vi "Paths to String with Commas.vi"(10 "Paths":string[](array[string])) -> (1 "Columns":string, 2 "Table":string)   [LabVIEW 2019, in "LV-Data.PGSQL.lvclass"]
uses:
  LV-Data.PGSQL.lvclass
  babc5d78-c446-43dc-b590-f0a1f3a79644.vi
panel:
  out "error out":errorcluster
  in  "error in":errorcluster
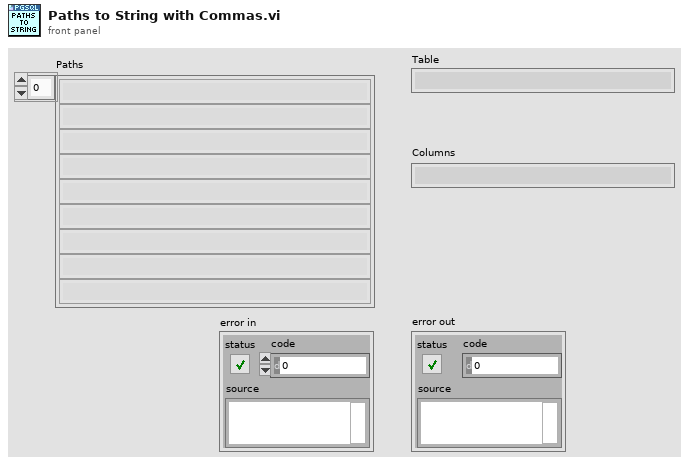
[diagram p1: front panel]
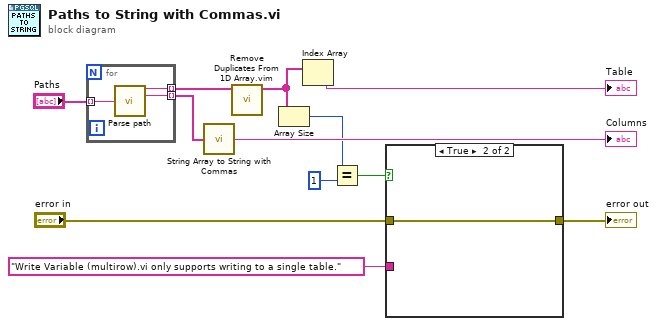
[diagram p0: block diagram]
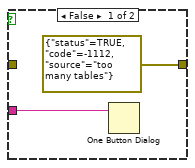
[diagram p2: hidden frame]
diagram:
  n1 = for {
    tunnel: [w14] -> w9 mode=indexing
    tunnel: "Paths" -> [w15] mode=indexing
    tunnel: [w13] -> w10 mode=indexing
    n2 = call "Parse path.vi"("PG Path"=w15) -> ("Table path"=w14:string, "Column path"=w13:string)  [unwired: 10 in, 3 out]
  }
  n3 = call "String Array to String with Commas.vi"("Array"=w10) -> ("String"=→"Columns":string)
  n4 = call "Remove Duplicates From 1D Array.vim"("array"=w9) -> ("array with duplicates removed"=w8:string[])  [unwired: 10 in]
  n5 = Array Size(array=w8) -> (size(s)=w5:i32)
  n6 = Index Array(array=w8) -> (element=→"Table":string)  [unwired: 1 in]
  n7 = Equal?(x=w5, y=1) -> (x = y?=w4:bool)
  n8 = case shown="True" w4 {
    tunnel: [errorcluster {"status"=TRUE, "code"=-1112, "source"="too many tables"} ("error in (no error)") w18] -> w3
    tunnel: "error in" -> [_ w18]
    tunnel: "Write Variable (multirow).vi only supports writing to a single table." ("message") -> [w16 _]
    frame False {
      n9 = One Button Dialog(message=w16) -> ()  [unwired: 1 in, 1 out]
    }
    frame True {
    }
  }
  "error out" <- w3
